vi "Thorlabs_CageRotator_dotNET.vi"(8 "error in (no error)":errorcluster, 11 "SerialNumber":string="27264338") -> (0 "error out":errorcluster)   [LabVIEW 2023]
doc: "This vi controls a Thorlabs Solenoid through a KCube KDC101 controller."
uses:
  C:/Users/Sebastien/Documents/GitHub/LABVIEW-Useful-codes/Device_control/Thorlabs_CageRotator_dotNET/dlls/Thorlabs.MotionControl.Controls.dll
  dlls/Thorlabs.MotionControl.Controls.dll
panel:
  in  "stop":bool
  in  "KCubeDCServoControl":refnum<k24>(container)
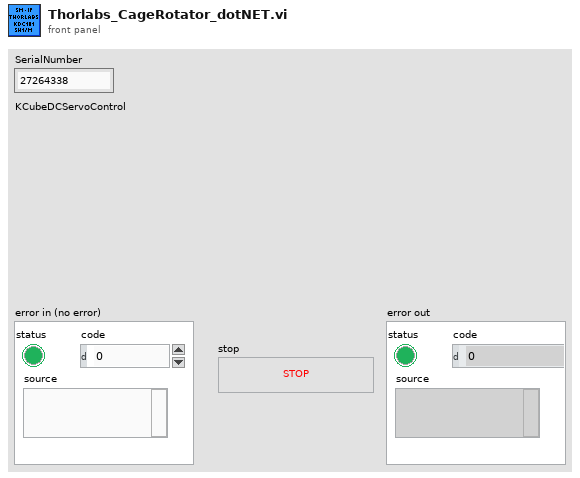
[diagram p1: front panel]
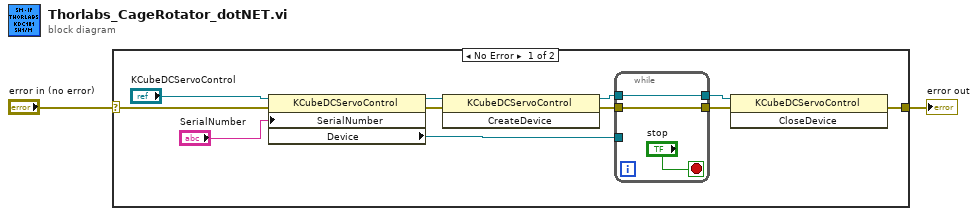
[diagram p0: block diagram]
diagram:
  n1 = case shown="No Error" "error in (no error)" {
    selector: "error in (no error)" -> [w4 w17]
    tunnel: [w5 w17] -> w2
    frame No Error {
      n2 = property class="KCubeDCServoControl"(reference="KCubeDCServoControl", error in=w4, "SerialNumber"="SerialNumber") -> (reference out=w11:refnum<k24>, error out=w6:errorcluster, "Device"=w3:refnum<k24>)
      n3 = invoke class="KCubeDCServoControl" method="CreateDevice"(reference=w11, error in=w6) -> (reference out=w10:refnum<k24>, error out=w7:errorcluster)  [unwired: 1 in, 1 out]
      n4 = while {
        tunnel: w10 -> [w15]
        tunnel: [w15] -> w9
        tunnel: [w14] -> w8
        tunnel: w7 -> [w14]
        tunnel: w3 -> [_]
        stop <- "stop" stop-if-true
      }
      n5 = invoke class="KCubeDCServoControl" method="CloseDevice"(reference=w9, error in=w8) -> (error out=w5:errorcluster)  [unwired: 1 in, 2 out]
    }
    frame Error {
    }
  }
  "error out" <- w2
